vi "AllThingsNotes.vi"(8 "Choice":string) -> (0 "Text":string, 3 "Array":string[](array[string]))   [LabVIEW 2022 SP3]
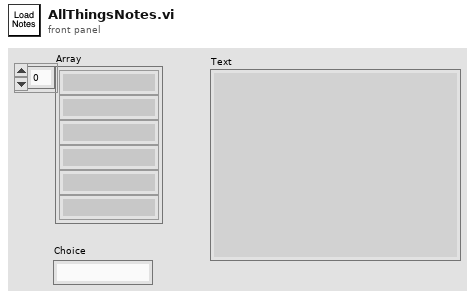
[diagram p1: front panel]
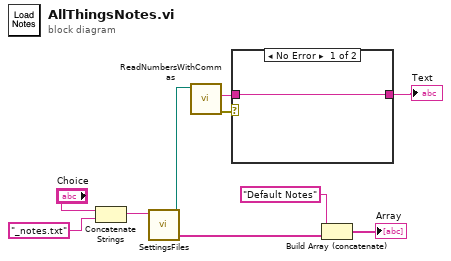
[diagram p0: block diagram]
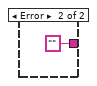
[diagram p2: hidden frame]
diagram:
  n1 = Concatenate Strings("Choice", "_notes.txt" ("pattern")) -> (w4:string)
  n2 = call "SettingsFiles.vi"("settings file name"=w4) -> ("filenames"=w1:string[], "file path"=w3:path)  [unwired: 9 in]
  n3 = call "ReadNumbersWithCommas.vi"("file (use dialog)"=w3) -> ("error out"=w6:errorcluster, "text"=w5:string)  [unwired: 7 in, 2 out]
  n4 = case shown="No Error" w6 {
    tunnel: [w11 ""] -> w7
    tunnel: w5 -> [w11 _]
    frame No Error {
    }
    frame Error {
    }
  }
  "Text" <- w7
  n5 = Build Array (concatenate)("Default Notes" ("string"), w1) -> (→"Array":string[])
